vi "Update Status.vi"(8 "error in (no error)":errorcluster, 11 "Transfer Group in":refnum<class "Transfer Group.lvclass">) -> (0 "error out":errorcluster, 3 "Transfer Group out":refnum<class "Transfer Group.lvclass">)   [LabVIEW 2021, in "DSF Core.lvlib" / "Transfer Group.lvclass"]
uses:
  Transfer Group.lvclass
  Transfer Group.lvclass/Transfer Group.ctl
  Timing/Timing.lvclass/Timing.ctl
  Performance/Performance.lvclass/Performance.ctl
  Status/Status Data.ctl
  <vilib>/NI/Memory Manager/Classes/Pointer/Pointer.lvclass/Pointer.ctl
  <vilib>/NI/Memory Manager/Classes/Pointer/Get Address.vi
  Status/Status Size.vi
  <vilib>/NI/Memory Manager/Classes/Pointer/Check Null Pointer.vi
  <vilib>/NI/Memory Manager/Classes/Pointer/Check Size.vi
  Timing/Get Iteration.vi
  <vilib>/NI/Memory Manager/Classes/Pointer/Errors.vi
  <vilib>/NI/Memory Manager/Classes/Pointer/Null Pointer.vi
  <vilib>/NI/Memory Manager/Classes/Pointer/Is Null.vi
  <vilib>/NI/Memory Manager/Classes/Pointer/Out of Bounds.vi
  <vilib>/NI/Memory Manager/Classes/Pointer/Get Size.vi
  <vilib>/NI/Memory Manager/Classes/Pointer/Create Error.vi
  <vilib>/NI/Memory Manager/VIs/Write String to Source.vi
  <vilib>/NI/Memory Manager/Classes/Pointer/Write Pointer Size to Error.vi
  <vilib>/NI/Memory Manager/VIs/Write Numeric to Source.vi
  <vilib>/NI/Memory Manager/VIs/Write Numeric Scalar to Source (Base10 U64).vi
  <vilib>/NI/Memory Manager/VIs/New Error Cluster.vi
  <vilib>/NI/Memory Manager/VIs/New Error Cluster (512B).vi
  <vilib>/NI/Memory Manager/VIs/Set Error Status.vi
  <vilib>/NI/Memory Manager/VIs/Set Error Code.vi
  <vilib>/NI/Memory Manager/VIs/Set Error Source.vi
  <vilib>/NI/Memory Manager/Constants/Constants.vi
  <vilib>/NI/Memory Manager/Constants/Library Name.vi
  <vilib>/NI/Memory Manager/Classes/Pointer/Pointer Error Info.vi
  <vilib>/NI/Memory Manager/Constants/Pointer Class Name.vi
  Status/Status Pointer.lvclass
  C:/Program Files/National Instruments/LabVIEW 2021/vi.lib/NI/Memory Manager/Classes/Pointer/Pointer.lvclass
  Performance/Performance.lvclass
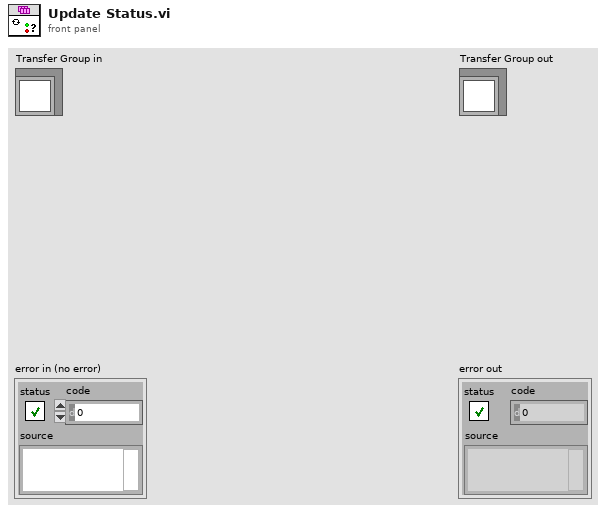
[diagram p1: front panel]
types:
  T1 = typedef "DSF Core.lvlib/Status Pointer.lvclass/Status Data.ctl" = cluster{"duration":u64, "period":u64, "iteration":u64, "late count":u64}
  T2 = typedef "DSF Core.lvlib/Timing Status Pointer.lvclass/Timing Status Data.ctl" = cluster{"rx start time":u32, "rx end time":u32, "tx start time":u32, "tx end time":u32, "cycle start time":u32, "cycle end time":u32, "prev start time":u32}
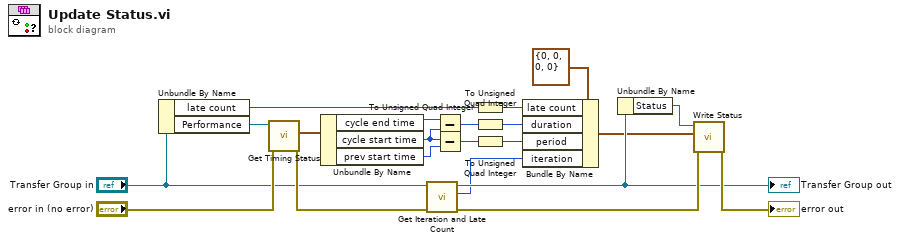
[diagram p0: block diagram]
diagram:
  n1 = Unbundle By Name("Transfer Group in") -> ("late count"=w17:i32, "Performance"=w16:refnum<class "Performance.lvclass">)
  n2 = call "Get Timing Status.vi"("error in (no error)"="error in (no error)", "Framework Performance in"=w16) -> ("error out"=w21:errorcluster, "timing status"=w12:T2)  [unwired: 7 in, 1 out]
  n3 = Unbundle By Name(w12) -> ("cycle end time"=w6:u32, "cycle start time"=w7:u32, "prev start time"=w11:u32)
  n4 = call "Get Iteration and Late Count.vi"("error in (no error)"=w21, "Transfer Group in"="Transfer Group in") -> ("error out"=w18:errorcluster, "iteration"=w4:u64, "Transfer Group out"=w9:refnum<class "Transfer Group.lvclass">)  [unwired: 6 in, 1 out]
  "Transfer Group out" <- w9
  n5 = Subtract(x=w6, y=w7) -> (x-y=w5:u32)
  n6 = Subtract(x=w7, y=w11) -> (x-y=w10:u32)
  n7 = To Unsigned Quad Integer(1:w17) -> (0:w3:u64)
  n8 = To Unsigned Quad Integer(1:w5) -> (0:w2:u64)
  n9 = To Unsigned Quad Integer(1:w10) -> (0:w1:u64)
  n10 = Bundle By Name(cluster=T1 {"duration"=0, "period"=0, "iteration"=0, "late count"=0} ("status"), "late count"=w3, "duration"=w2, "period"=w1, "iteration"=w4) -> (w8:T1)
  n11 = Unbundle By Name(w9) -> ("Status"=w13:refnum<class "Status Pointer.lvclass">)
  n12 = call "Write Status.vi"("error in (no error)"=w18, "status"=w8, "status pointer in"=w13) -> ("error out"=→"error out":errorcluster)  [unwired: 7 in, 1 out]
